vi "DG535.set C mode.vi"(0 "i ref in":refnum<vi>, 7 "mode":i32(ring) items=["TTL", "NIM", "ECL", "VAR"], 11 "error in":errorcluster) -> (4 "i ref out":refnum<vi>, 15 "error out":errorcluster)   [LabVIEW 2014, in "DG535.lvlib"]
uses:
  DG535.lvlib
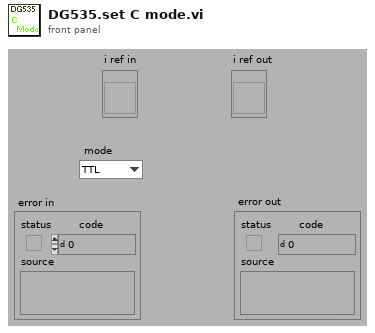
[diagram p1: front panel]
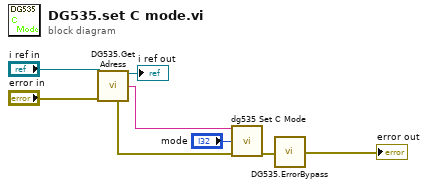
[diagram p0: block diagram]
diagram:
  n1 = call "DG535.Get Adress.vi"("i ref in"="i ref in", "error in (no error)"="error in") -> ("i ref out"=→"i ref out":refnum<vi>, "address"=w7:string, "error out"=w6:errorcluster)  [unwired: 10 in, 1 out]
  n2 = call "dg535 Set C Mode.vi"("address string"=w7, "mode"="mode", "error in"=w6) -> ("error out"=w8:errorcluster)  [unwired: 12 in]
  n3 = call "DG535.ErrorBypass.vi"("error in (no error)"=w8) -> ("error out"=→"error out":errorcluster)  [unwired: 14 in]
